vi "onListenForNewConnection.vi"(8 "error in (no error)":errorcluster, 9 "timeout (ms)":i32=2000, 11 "Listener":refnum<class "TCPConnection.lvclass">) -> (0 "error out":errorcluster, 1 "New connection":bool, 2 "timed out":bool, 3 "New Connection":refnum<class "Connection.lvclass">)   [LabVIEW 2013, in "MQTT_TCP.lvlib" / "TCPConnection.lvclass"]
uses:
  TCPConnection.lvclass
  <vilib>/LabVIEW Open Source Project/MQTT Connection/MQTT_Connection/Connection/Connection.lvclass
  TCPConnection.lvclass/TCPConnection.ctl
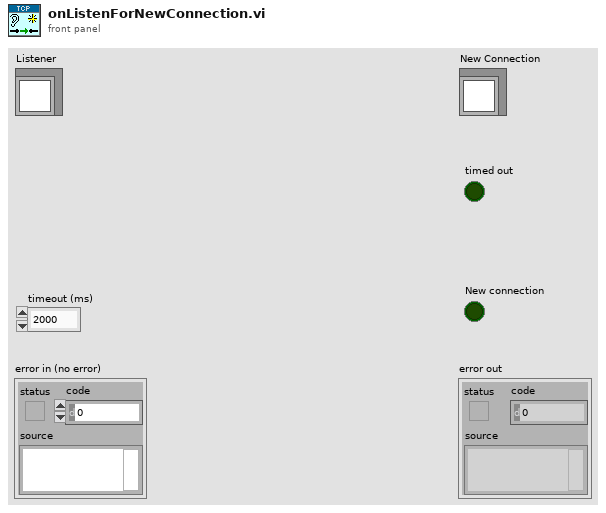
[diagram p1: front panel]
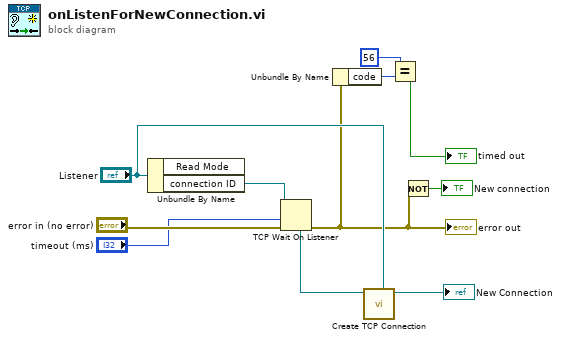
[diagram p0: block diagram]
diagram:
  n1 = Unbundle By Name("Listener") -> ("connection ID"=w9:refnum<k5>)  [unwired: 1 out]
  n2 = TCP Wait On Listener(8:"error in (no error)", 9:"timeout (ms)", 11:w9) -> (0:w4:errorcluster, 4:w7:refnum<k5>)  [unwired: 1 in, 3 out]
  "error out" <- w4
  n3 = Unbundle By Name(w4) -> ("code"=w3:i32)
  n4 = call "Create TCP Connection.vi"("TCPConnection in"="Listener", "connection ID"=w7) -> ("TCPConnection out"=→"New Connection":refnum<class "TCPConnection.lvclass">)  [unwired: 8 in, 1 out]
  n5 = Equal?(x=56, y=w3) -> (x = y?=→"timed out":bool)
  n6 = Not(x=w4) -> (.not. x?=→"New connection":bool)
